vi "MSG to Target Cannot be Sent --error.vi"() -> (0 "error out":errorcluster)   [LabVIEW 2021, in "Host Interpreter.lvlib"]
doc: "Outputs an error cluster containing a custom error code indicating the module is not running.\n_____\nBased on DQMH Dev Tools: Project Template 7.1.2.1547."
uses:
  Host Interpreter.lvlib
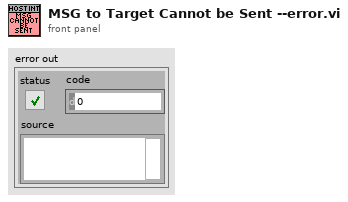
[diagram p1: front panel]
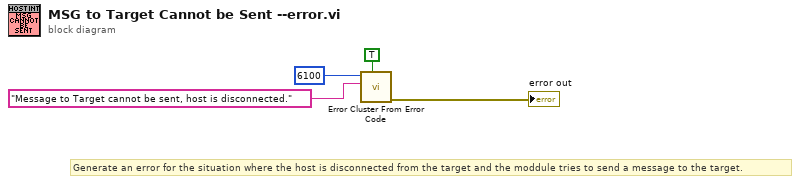
[diagram p0: block diagram]
diagram:
  # "Generate an error for the situation where the host is disconnected from the target and the moddule tries to send a message to the target."
  n1 = call <vilib>:"Error Cluster From Error Code.vi"("show call chain? (False)"=TRUE, "error message (\"\")"="Message to Target cannot be sent, host is disconnected.", "error code (0)"=6100) -> ("error out"=→"error out":errorcluster)  [unwired: 6 in]
